vi "example 4b - child.vi"() -> ()   [LabVIEW 2020]
panel:
  in  "Multicolumn Listbox":i32(listbox)
  in  "Listbox":i32(listbox)
  in  "Tree":string[](tree)
  in  "String":string
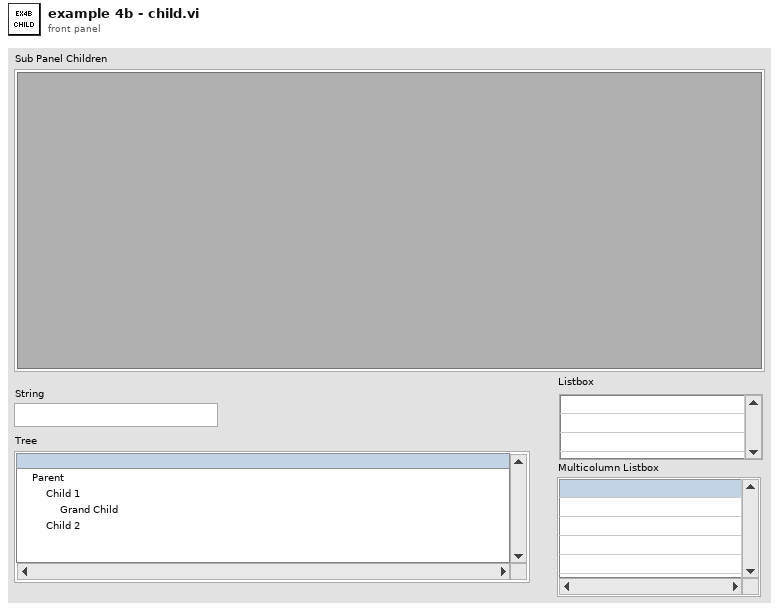
[diagram p1: front panel]
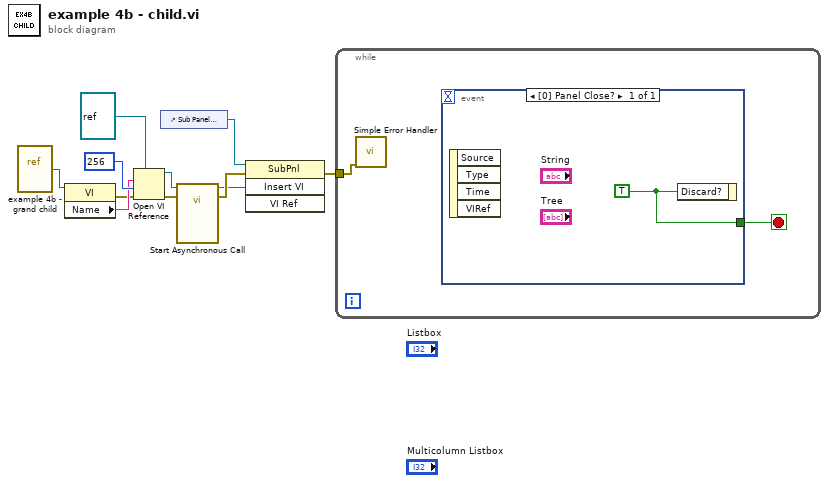
[diagram p0: block diagram]
diagram:
  n1 = vi-ref "example 4b - grand child.vi"() -> (w7:refnum<vi>)
  n2 = property class="VI"(reference=w7) -> (error out=w5:errorcluster, "Name"=w6:string)  [unwired: 1 in, 1 out]
  n3 = Open VI Reference(type specifier VI Refnum (for type only)=refnum<vi> refnum, vi path=w6, options=256 ("call and forget"), error in (no error)=w5) -> (vi reference=w9:refnum<vi>, error out=w8:errorcluster)  [unwired: 2 in]
  n4 = control-ref of="Sub Panel Children"() -> (w1:refnum<vi>)
  n5 = call-by-ref "Start Asynchronous Call"(reference=w9, error in=w8) -> (reference out=w3:refnum<vi>, error out=w4:errorcluster)  [unwired: 12 in]
  n6 = invoke on="Invoke Node" class="SubPnl" method="Insert VI"(reference=w1, error in=w4, "VI Ref"=w3) -> (error out=w2:errorcluster)  [unwired: 1 in, 3 out]
  n7 = while {
    tunnel: w2 -> [w12]
    stop <- w13 stop-if-true
    n8 = call <vilib>:"Simple Error Handler.vi"("error in (no error)"=w12) -> ()  [unwired: 4 in, 5 out]
    n9 = event shown="[0] Panel Close?" {
      selector: _ -> [_]
      dyn-events: _ -> [_]
      timeout: _ -> [_]
      tunnel: [w14] -> w13
      event Panel Close? {
        w14 = TRUE
        n10 = event-data() -> ()  [unwired: 1 in, 4 out]
        n11 = event-data("Discard?"=w14) -> ()  [unwired: 1 in, 1 out]
      }
    }
  }
